vi "LIA Vrms2 to dBm.vi"(11 "Power Spectrum / PSD in":cluster{"f0":dbl, "df":dbl, "magnitude":dbl[]}) -> (3 "Power Spectrum / PSD out":cluster{"f0":dbl, "df":dbl, "magnitude":dbl[]})   [LabVIEW 2018]
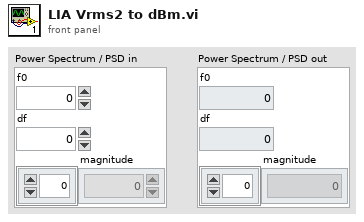
[diagram p1: front panel]
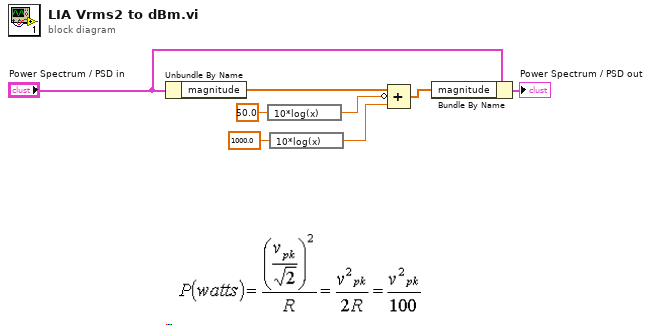
[diagram p0: block diagram]
diagram:
  n1 = Unbundle By Name("Power Spectrum / PSD in") -> ("magnitude"=w2:dbl[])
  n2 = expression code="10*log(x)"(50.0) -> (w5:dbl)
  n3 = expression code="10*log(x)"(1000.0) -> (w8:dbl)
  n4 = Compound Arithmetic op=ADD(w2, invert w5, w8) -> (w4:dbl[])
  n5 = Bundle By Name(cluster="Power Spectrum / PSD in", "magnitude"=w4) -> (→"Power Spectrum / PSD out":cluster{"f0":dbl, "df":dbl, "magnitude":dbl[]})
